vi "3. Copy Image Symmetry And Merge.vi"() -> ()   [LabVIEW 2019]
doc: "c 2020 ReMiSYS All rights reserved."
uses:
  <vilib>/vision/NI_Vision_Development_Module.lvlib
panel:
  in  "Stop (F)":bool
  out "final":T1(plugin-control)
  out "sym":T1(plugin-control)
  out "ori":T1(plugin-control)
  # "c 2022 ReMiSYS All rights reserved."
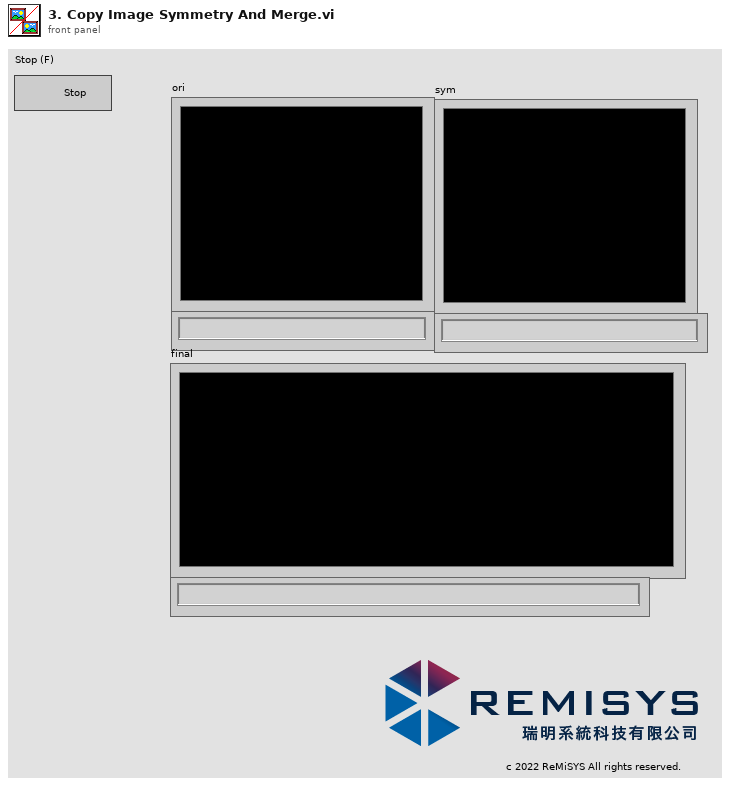
[diagram p1: front panel]
types:
  T1 = typedef "IMAQ Image.ctl" = refnum<image>
  T2 = typedef "Image Type" = u32
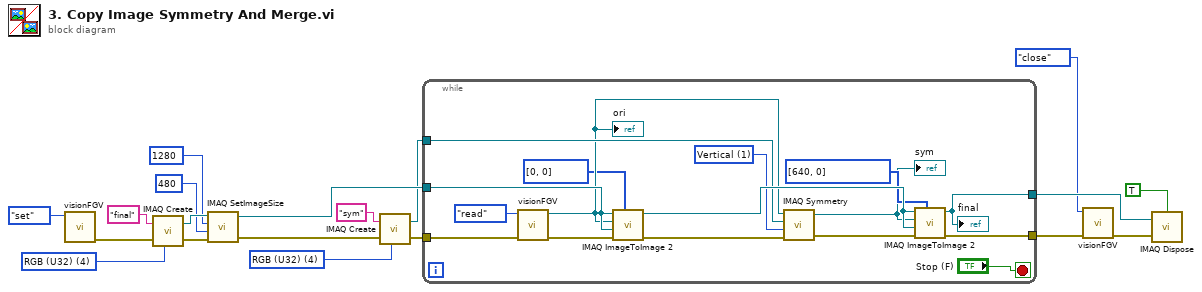
[diagram p0: block diagram]
diagram:
  w9 = T2 4 items=["Grayscale (U8)", "Grayscale (I16)", "Grayscale (SGL)", "Complex (CSG)", "RGB (U32)", "HSL (U32)", "RGB (U64)", "Grayscale (U16)"] ("Image Type")
  w14 = T2 4 items=["Grayscale (U8)", "Grayscale (I16)", "Grayscale (SGL)", "Complex (CSG)", "RGB (U32)", "HSL (U32)", "RGB (U64)", "Grayscale (U16)"] ("Image Type")
  n1 = call "visionFGV.vi"("Function"=enum16{"set", "read", "close"}."set") -> ("error out"=w3:errorcluster)  [unwired: 9 in, 1 out]
  n2 = call "IMAQ Create"("Image Name"="final", "Image Type"=w14, "error in (no error)"=w3) -> ("New Image"=w16:T1, "error out"=w8:errorcluster)  [unwired: 2 in]
  n3 = call "IMAQ SetImageSize"("error in (no error)"=w8, "Y Resolution"=480, "X Resolution"=1280, "Image"=w16) -> ("error out"=w7:errorcluster, "Image Out"=w15:T1)  [unwired: 1 in]
  n4 = call "IMAQ Create"("Image Name"="sym", "Image Type"=w9, "error in (no error)"=w7) -> ("New Image"=w13:T1, "error out"=w6:errorcluster)  [unwired: 2 in]
  n5 = while {
    tunnel: w15 -> [w35]
    tunnel: w13 -> [w30]
    tunnel: [w27] -> w12
    tunnel: w6 -> [w24]
    tunnel: [w22] -> w5
    stop <- "Stop (F)" stop-if-true
    w31 = u32 1 items=["Horizontal", "Vertical", "Central", "1st Diagonal", "2nd Diagonal"] ("Type of Symmetry")
    n6 = call "visionFGV.vi"("Error In"=w24, "Function"=enum16{"set", "read", "close"}."read") -> ("error out"=w23:errorcluster, "Image Out fgv"=w29:T1)  [unwired: 8 in]
    "ori" <- w29
    n7 = call "IMAQ ImageToImage 2"("Offset Left/Top"=i32[] [0, 0], "error in (no error)"=w23, "Image Dst"=w35, "Image Src (Small)"=w29, "Image Src (Large)"=w35) -> ("error out"=w26:errorcluster, "Image Dst Out"=w34:T1)  [unwired: 5 in]
    n8 = call "IMAQ Symmetry"("error in (no error)"=w26, "Type of Symmetry"=w31, "Image Dst"=w30, "Image Src"=w29) -> ("error out"=w25:errorcluster, "Image Dst Out"=w32:T1)  [unwired: 1 in]
    "sym" <- w32
    n9 = call "IMAQ ImageToImage 2"("Offset Left/Top"=i32[] [640, 0], "error in (no error)"=w25, "Image Dst"=w34, "Image Src (Small)"=w32, "Image Src (Large)"=w34) -> ("error out"=w22:errorcluster, "Image Dst Out"=w27:T1)  [unwired: 5 in]
    "final" <- w27
  }
  n10 = call "visionFGV.vi"("Error In"=w5, "Function"=enum16{"set", "read", "close"}."close") -> ("error out"=w2:errorcluster)  [unwired: 8 in, 1 out]
  n11 = call "IMAQ Dispose"("All Images? (No)"=TRUE, "Image"=w12, "error in (no error)"=w2) -> ()  [unwired: 3 in, 1 out]
